vi "Get Traverse Names.vi"(2 "Traverse name":string, 3 "Traverse\nSetup\nFolder":path) -> (0 "error out":errorcluster, 1 "Traverse Names":string[](array[string]))   [LabVIEW 2022 SP3]
uses:
  Globals/Constants_global.vi
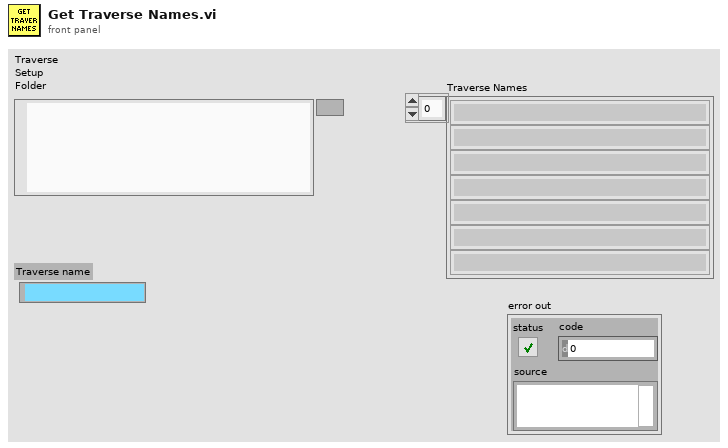
[diagram p1: front panel]
types:
  T1 = enum16{"Zero or one", "One", "Zero or more", "One or more"}
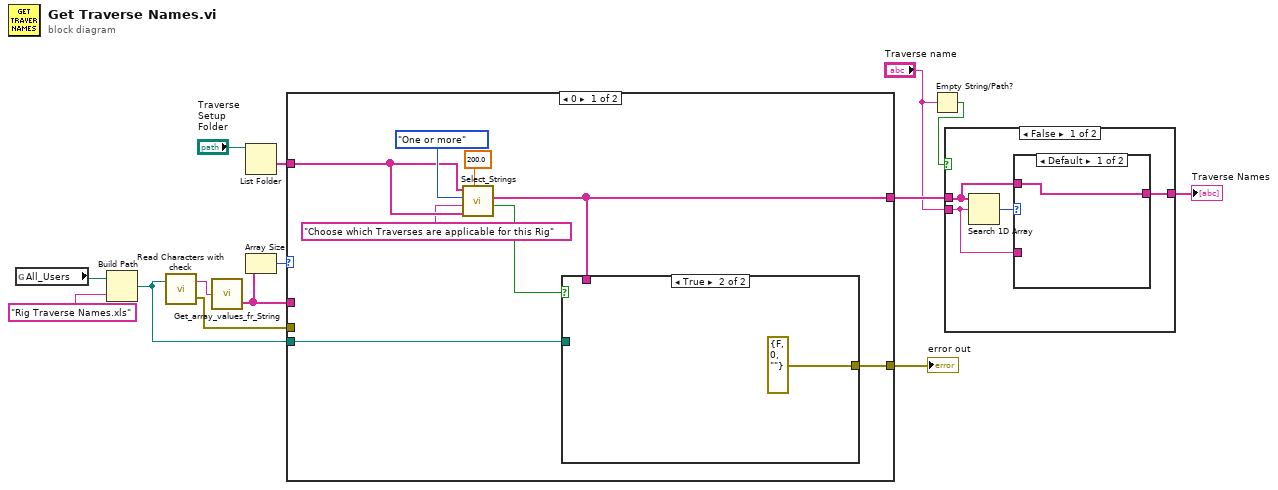
[diagram p0: block diagram]
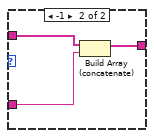
[diagram p2: hidden frame]
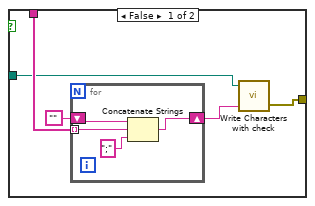
[diagram p4: hidden frame]
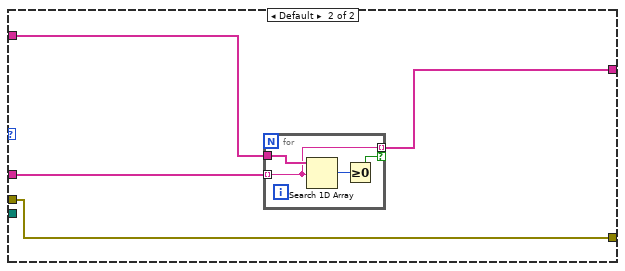
[diagram p5: hidden frame]
diagram:
  n1 = global read "Constants_global.vi" "All_Users"() -> (w11:path)
  n2 = Build Path(base path=w11, name or relative path="Rig Traverse Names.xls") -> (appended path=w7:path)
  n3 = call "Read Characters with check.vi"("file (use dialog)"=w7) -> ("error out"=w5:errorcluster, "Read String"=w6:string)  [unwired: 1 in]
  n4 = call "Get_array_values_fr_String.vi"("String Value"=w6) -> ("String array"=w13:string[])  [unwired: 1 out]
  n5 = List Folder(path="Traverse\nSetup\nFolder") -> (folder names=w12:string[])  [unwired: 1 in, 5 out]
  n6 = Array Size(array=w13) -> (size(s)=w14:i32)
  n7 = case shown="0" w14 {
    tunnel: w12 -> [w21 w36]
    tunnel: w13 -> [_ w35]
    tunnel: [w17 w34] -> w2
    tunnel: w7 -> [w16 _]
    tunnel: [w15 w33] -> w8
    tunnel: w5 -> [_ w33]
    frame 0 {
      n8 = call "Select_Strings.vi"("Timeout (s)"=200.0, "Available Ch names"=w21, "Message"="Choose which Traverses are applicable for this Rig", "Selector mode"=T1."One or more", "Desired Ch names (in)"=w21) -> ("Cancel"=w18:bool, "Selected Channel Names"=w17:string[])  [unwired: 1 in, 1 out]
      n9 = case shown="True" w18 {
        tunnel: w17 -> [w27 _]
        tunnel: w16 -> [w25 _]
        tunnel: [w23 errorcluster {"status"=FALSE, "code"=0, "source"=""} ("error out")] -> w15
        frame False {
          n10 = for {
            shift-right: [w30] -> w24
            shift-left: "" -> [w31]
            tunnel: w27 -> [w29] mode=indexing
            n11 = Concatenate Strings(w31, w29, ";") -> (w30:string)
          }
          n12 = call "Write Characters with check.vi"("String to Write"=w24, "file (use dialog)"=w25) -> ("error out"=w23:errorcluster)  [unwired: 2 in]
        }
        frame True {
        }
      }
    }
    frame Default {
      n13 = for {
        tunnel: w35 -> [w38] mode=indexing
        tunnel: w36 -> [w40]
        tunnel: [w38] -> w34 mode=indexing if=w37
        n14 = Search 1D Array(1D array=w40, element=w38) -> (index of element=w39:i32)  [unwired: 1 in]
        n15 = Greater Or Equal To 0?(x=w39) -> (x >= 0?=w37:bool)
      }
    }
  }
  "error out" <- w8
  n16 = Empty String/Path?(string/path="Traverse name") -> (empty?=w4:bool)
  n17 = case shown="False" w4 {
    tunnel: [w43 w49] -> w3
    tunnel: w2 -> [w42 w49]
    tunnel: "Traverse name" -> [w41 _]
    frame False {
      n18 = Search 1D Array(1D array=w42, element=w41) -> (index of element=w44:i32)  [unwired: 1 out]
      n19 = case shown="Default" w44 {
        tunnel: [w45 w47] -> w43
        tunnel: w42 -> [w45 w48]
        tunnel: w41 -> [_ w46]
        frame Default {
        }
        frame -1 {
          n20 = Build Array (concatenate)(w48, w46) -> (w47:string[])
        }
      }
    }
    frame True {
    }
  }
  "Traverse Names" <- w3
